vi "Clear IP.vi"(8 "error in (no error)":errorcluster, 11 "Analog Replay in":refnum<class "Analog Replay.lvclass">) -> (0 "error out":errorcluster)   [LabVIEW 2013, in "Analog Replay.lvclass"]
uses:
  Analog Replay.lvclass
  Engine Simulation IP.lvclass
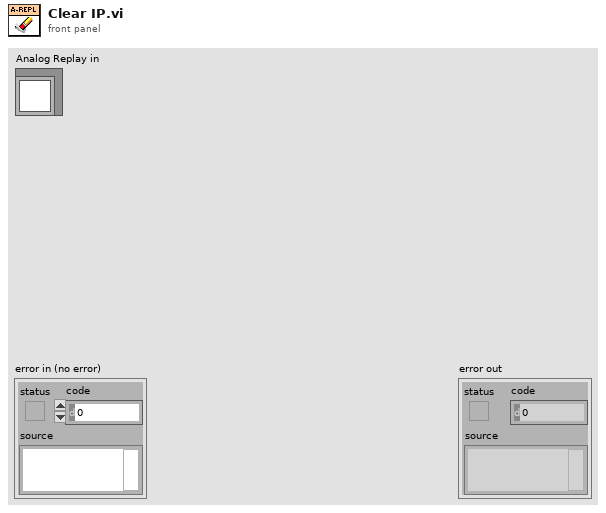
[diagram p1: front panel]
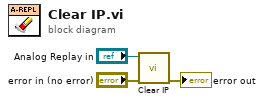
[diagram p0: block diagram]
diagram:
  n1 = call-parent "Clear IP.vi"("error in (no error)"="error in (no error)", "Engine Simulation IP in"="Analog Replay in") -> ("error out"=→"error out":errorcluster)  [unwired: 9 in]
